vi "UpdateMDF.vi"(8 "Index":i32, 11 "Where-to-Where In":T1(array[cluster])=[{"Waypoint Lat."=0.0, "Waypoint Lon."=0.0, "Current Lat."=0.0, "Current Lon. "=0.0, "Current Velocity"=0.0, "Current Heading"=0.0, "Desired Velocity"=0.0, "Mode"=enum."Traverse the O", "Status"=enum."Current"}]) -> (3 "Where-to-Where updated":T1(array[cluster])=[{"Waypoint Lat."=0.0, "Waypoint Lon."=0.0, "Current Lat."=0.0, "Current Lon. "=0.0, "Current Velocity"=0.0, "Current Heading"=0.0, "Desired Velocity"=0.0, "Mode"=enum."Traverse the O", "Status"=enum."Current"}])   [LabVIEW 2010]
doc: "This VI updates the status control in the MDF cluster"
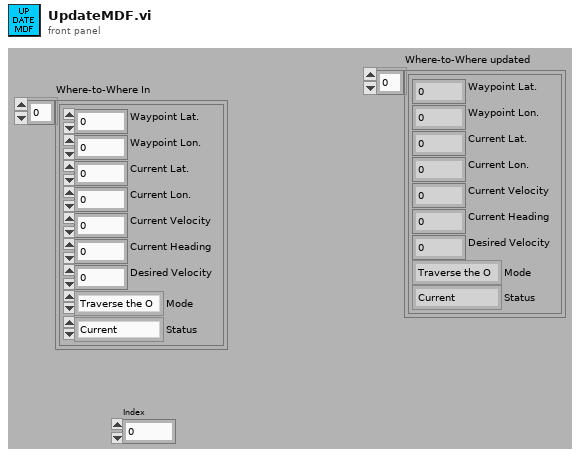
[diagram p1: front panel]
types:
  T1 = cluster{"Waypoint Lat.":dbl, "Waypoint Lon.":dbl, "Current Lat.":dbl, "Current Lon. ":dbl, "Current Velocity":dbl, "Current Heading":dbl, "Desired Velocity":dbl, "Mode":enum16{"Traverse the O"}, "Status":enum16{"Current", "Future", "Past"}}[]
  T2 = cluster{"Waypoint Lat.":dbl, "Waypoint Lon.":dbl, "Current Lat.":dbl, "Current Lon. ":dbl, "Current Velocity":dbl, "Current Heading":dbl, "Desired Velocity":dbl, "Mode":enum16{"Traverse the O"}, "Status":enum16{"Current", "Future", "Past"}}
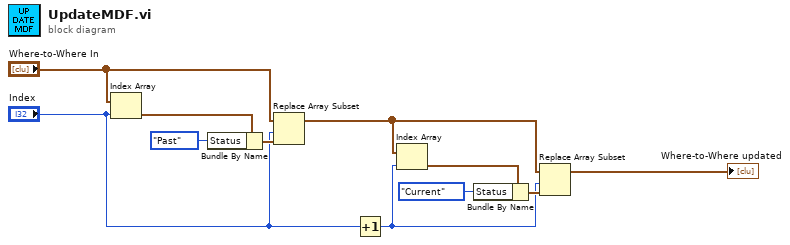
[diagram p0: block diagram]
diagram:
  n1 = Index Array "Index Array"(array="Where-to-Where In", index="Index") -> (element=w11:T2)
  n2 = Bundle By Name(cluster=w11, "Status"=enum16{"Current", "Future", "Past"}."Past") -> (w10:T2)
  n3 = Replace Array Subset "Replace Array Subset"(array="Where-to-Where In", new element=w10, index="Index") -> (w8:T1)
  n4 = Increment(x="Index") -> (x+1=w5:i32)
  n5 = Index Array "Index Array"(array=w8, index=w5) -> (element=w7:T2)
  n6 = Bundle By Name(cluster=w7, "Status"=enum16{"Current", "Future", "Past"}."Current") -> (w6:T2)
  n7 = Replace Array Subset "Replace Array Subset"(array=w8, new element=w6, index=w5) -> (→"Where-to-Where updated":T1)
